vi "Parse Clusters.vi"(8 "error in (no error)":errorcluster, 9 "CLuster Ring":refnum<vi>, 10 "Interface Type":u16(ring)=1 items=["CAN", "FlexRay"], 11 "XNET Database":refnum<k21>="nixnet_example") -> (0 "error out":errorcluster)   [LabVIEW 2009]
doc: "This VI parses the clusters read in a database according to the protocol that is selected. This is done to make sure a FlexRay cluster is NOT selected with a CAN interface."
uses:
  Program Files/National Instruments/LabVIEW 2009/resource/objmgr/xnet.rc
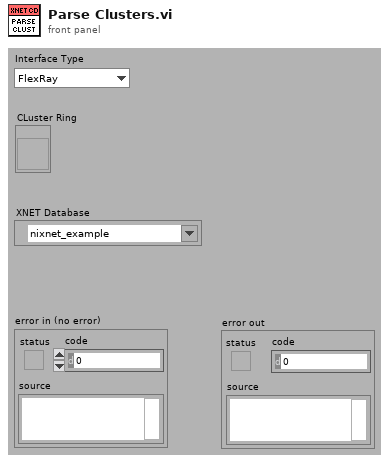
[diagram p1: front panel]
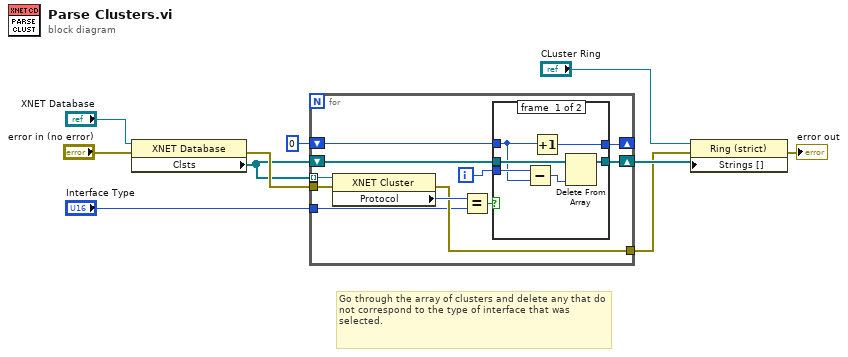
[diagram p0: block diagram]
diagram:
  # "Go through the array of clusters and delete any that do not correspond to the type of interface that was selected."
  n1 = property class="XNET Database"(reference="XNET Database", error in="error in (no error)") -> (error out=w9:errorcluster, "Clsts"=w8:refnum<k21>[])  [unwired: 1 out]
  n2 = for {
    tunnel: w8 -> [w21] mode=indexing
    tunnel: w9 -> [w20]
    shift-right: [w16] -> w6
    shift-left: w8 -> [w18]
    shift-right: [w13] -> _
    shift-left: 0 -> [w14]
    tunnel: [w12] -> w5
    tunnel: "Interface Type" -> [w11]
    i -> [w15]
    n3 = property class="XNET Cluster"(reference=w21, error in=w20) -> (error out=w12:errorcluster, "Protocol"=w19:u32)  [unwired: 1 out]
    n4 = Equal?(x=w19, y=w11) -> (x = y?=w17:bool)
    n5 = case shown="False" w17 {
      tunnel: w18 -> [w27 w29]
      tunnel: [w26 w29] -> w16
      tunnel: w15 -> [w23 _]
      tunnel: w14 -> [w22 w28]
      tunnel: [w24 w28] -> w13
      frame #0 {
        n6 = Subtract(x=w23, y=w22) -> (x-y=w25:i32)
        n7 = Increment(x=w22) -> (x+1=w24:i32)
        n8 = Delete From Array(array=w27, index=w25) -> (array with subset deleted=w26:refnum<k21>[])  [unwired: 1 in, 1 out]
      }
      frame #1 {
      }
    }
  }
  n9 = property on="Property Node" class="Ring (strict)"(reference="CLuster Ring", error in=w5, "Strings []"=w6) -> (error out=→"error out":errorcluster)  [unwired: 1 out]
